vi "Destroy.vi"(0 "reference in":refnum<class "MyG#SubClass.lvclass">, 5 "error in (no error)":errorcluster) -> (14 "reference out":refnum<class "MyG#SubClass.lvclass">, 19 "error out":errorcluster)   [LabVIEW 2017, in "MyG#SubClass.lvclass"]
doc: "Destructor."
uses:
  MyG#SubClass.lvclass
  MyG#Class_class/MyG#Class.lvclass
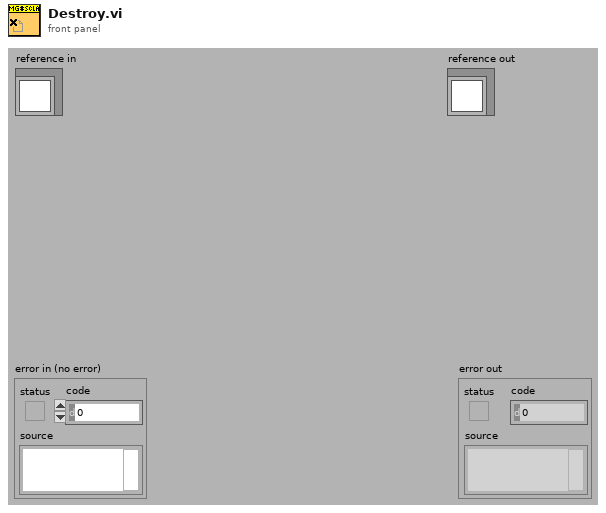
[diagram p1: front panel]
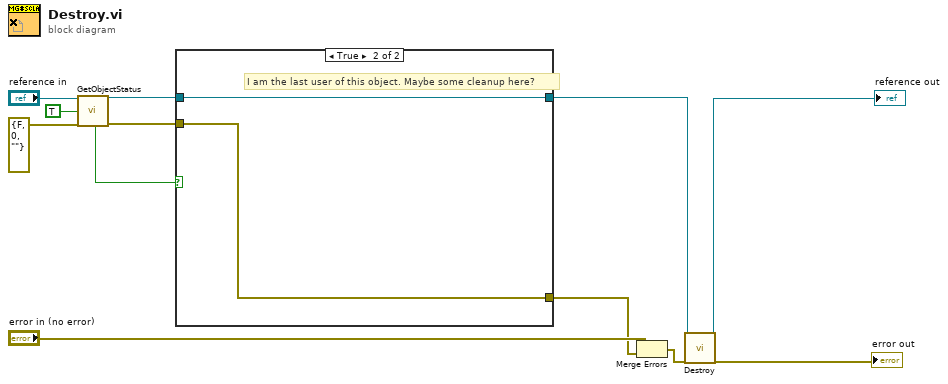
[diagram p0: block diagram]
diagram:
  n1 = call-dynamic "GetObjectStatus.vi"("reference in"="reference in", "simple info (F)"=TRUE ("simple info"), "error in (no error)"=errorcluster {"status"=FALSE, "code"=0, "source"=""}) -> ("last user"=w1:bool, "reference out"=w5:refnum<class "MyG#SubClass.lvclass">, "error out"=w6:errorcluster)  [unwired: 5 in, 9 out]
  n2 = case shown="True" w1 {
    tunnel: [w13 w15] -> w7
    tunnel: w6 -> [w13 w15]
    tunnel: w5 -> [w14 w16]
    tunnel: [w14 w16] -> w4
    frame False {
    }
    frame True {
      # "I am the last user of this object. Maybe some cleanup here?"
    }
  }
  n3 = Merge Errors("error in (no error)", w7) -> (w11:errorcluster)
  n4 = call-parent "Destroy.vi"("reference in"=w4, "error in (no error)"=w11) -> ("reference out"=→"reference out":refnum<class "MyG#SubClass.lvclass">, "error out"=→"error out":errorcluster)  [unwired: 16 in]
